vi "Scan1762ARP.vi"() -> ()   [LabVIEW 2012]
uses:
  <vilib>/Utility/file.llb/Write To Spreadsheet File (DBL).vi
panel:
  in  "1762 Sweep freq Span(Hz)":dbl=100000.0
  out "DARK?":i32(graph)=41
  out "Counts":i32=41
  out "DARK?":bool
  out "PMT Counts":i32(graph)=29
  in  "PMT sample time":dbl=0.02
  out "Counts after 1762":i32=29
  out "OuterLoop":i32
  out "InnerLoop":i32=23
  out "Bright Events":dbl=71.0
  in  "Discriminator Level\n (Bright/Dark)":i32=12
  in  "1762 Sweep time (ms)":i32=20
  in  "Comment":string="SPAOM, DPAOM = 83 MHz"
  in  "Rerun BG Every\nnth freq point":dbl=2.0
  in  "PMT sample time":dbl=0.02
  out "Counts finding bright ion":dbl=41.0
  in  "BG Cutoff Limit":dbl=25.0
  in  "Runs per data point":dbl=100.0
  in  "Low Freq":dbl(slide)=82000000.0 min=50000000.0 max=120000000.0 step=1000.0 scale=75000000.0..90000000.0 scale format="%#.5f"
  in  "High Freq":dbl(slide)=85000000.0 min=50000000.0 max=120000000.0 step=1000.0 scale=80000000.0..90000000.0 scale format="%#.0f"
  out "Cur Freq":dbl=85000000.0 format="%#_8f"
  out "Path":path=path "c:/data/1762 Scans/2014-06-11_11-58-27_1762scanWithPumping.txt"
  out "Frequency Scan":cluster{dbl, dbl}[](graph)=[{88000000.0, 1.29}, {87600000.0, 1.0}, {87200000.0, 1.0}, {86800000.0, 1.0}, {86400000.0, 1.0}, {86000000.0, 0.99}, {85600000.0, 1.0}, {85200000.0, 1.0}, {84800000.0, 1.0}, {84400000.0, 0.99}, {84000000.0, 1.0}, {83600000.0, 1.0}, {83200000.0, 0.99}, {82800000.0, 0.88}, {82400000.0, 1.0}, {82000000.0, 1.0}]
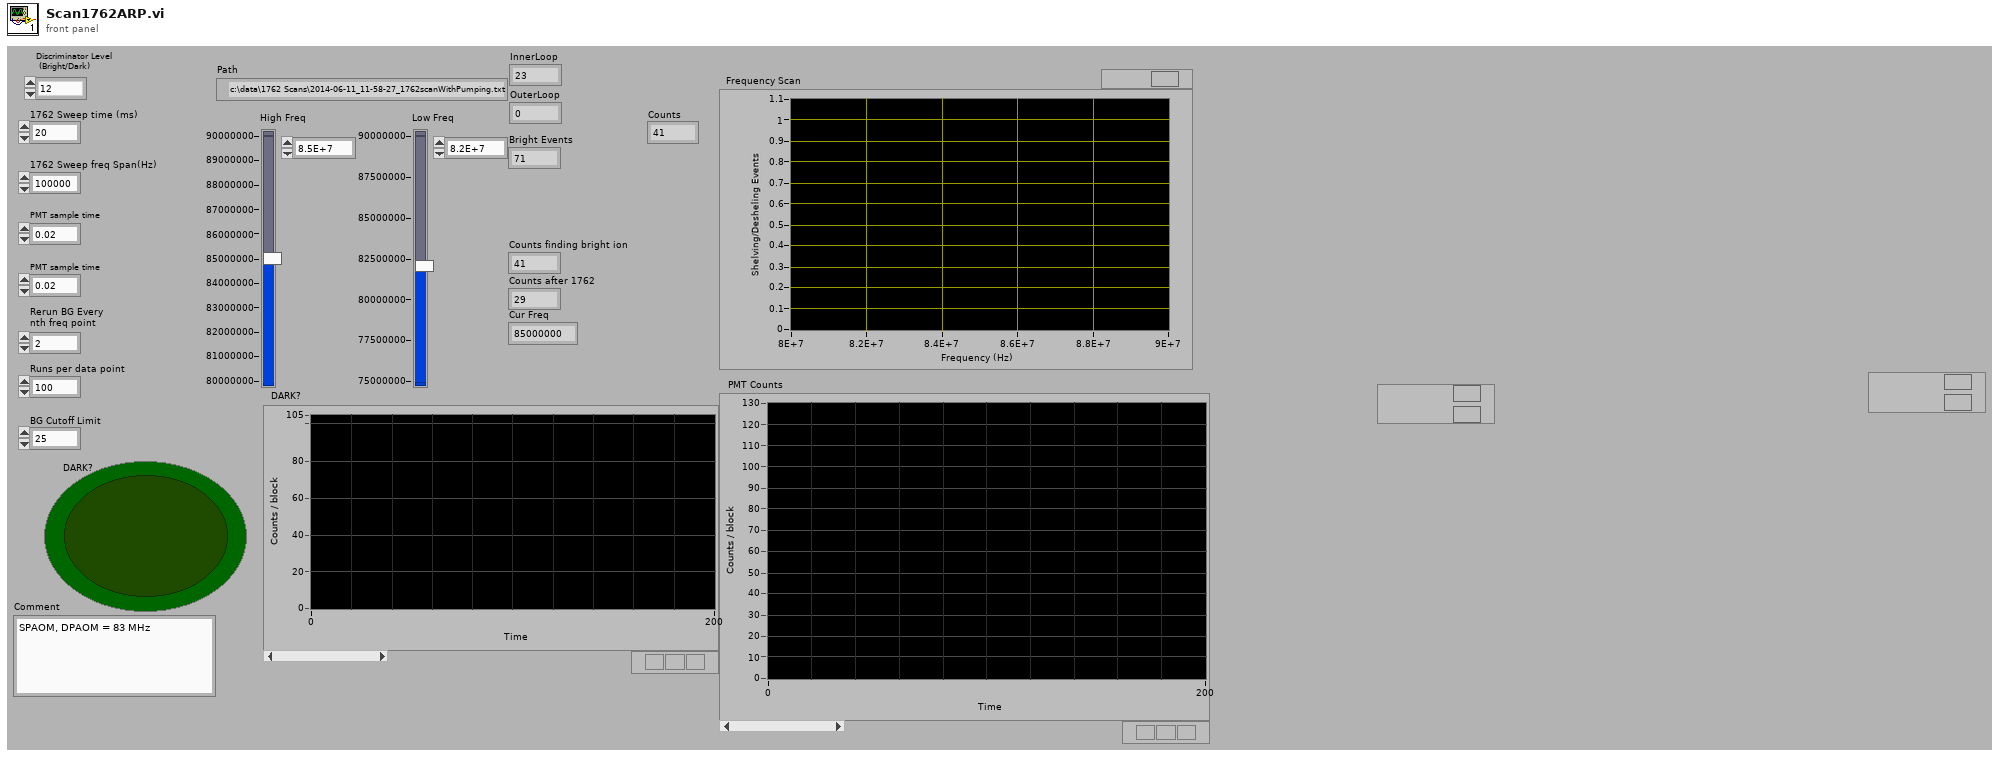
[diagram p1: front panel]
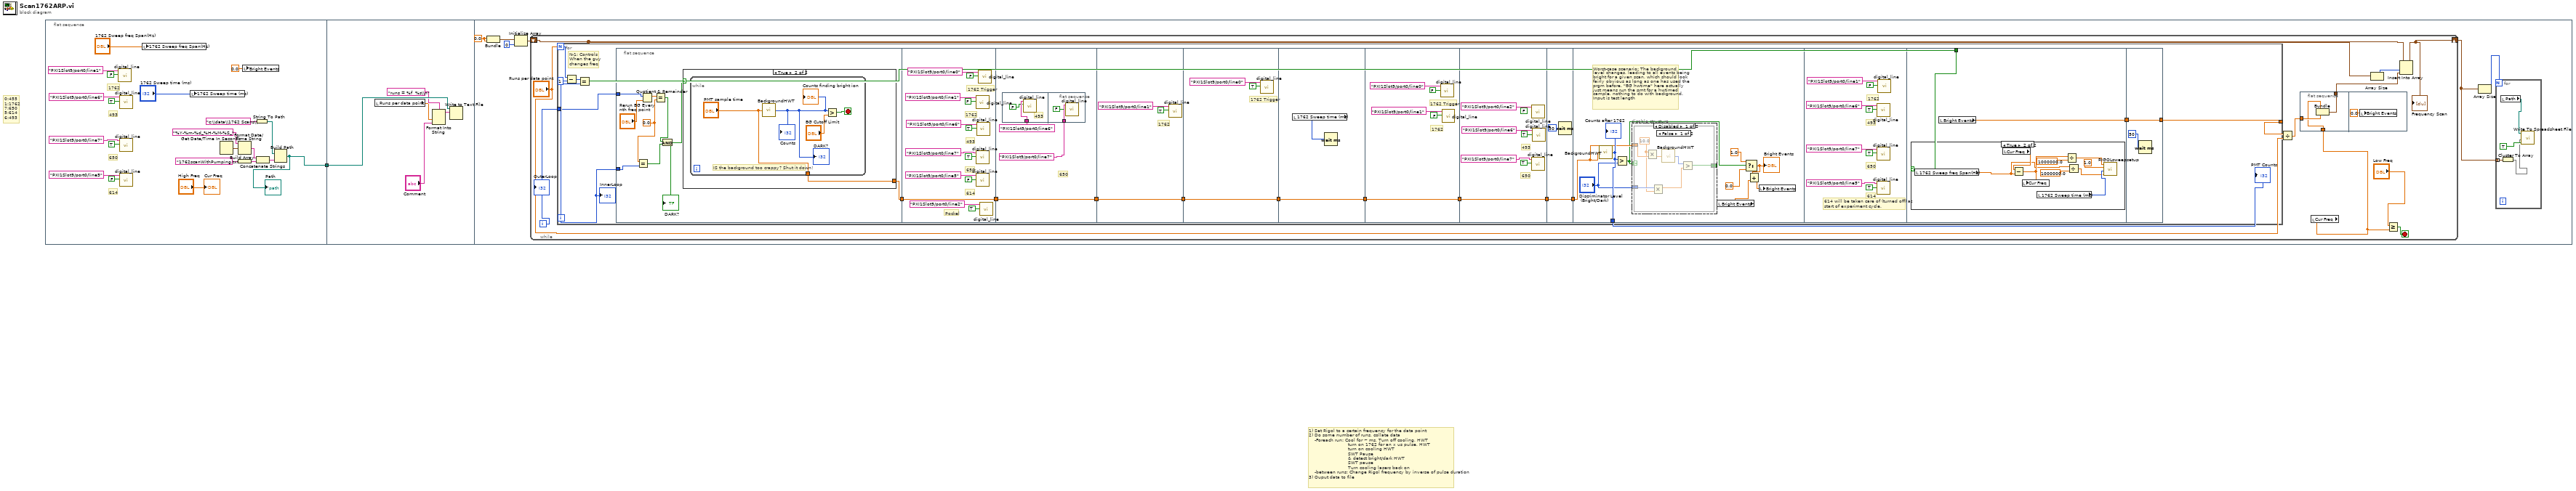
[diagram p0: block diagram]
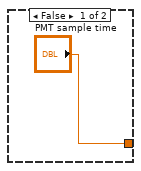
[diagram p2: hidden frame]
diagram:
  # "0:455\n1:1762\n7:650\n5:614\n6:493"
  # "1) Set Rigol to a certain frequency for the data point\n2) Do some number of runs, collate data\n    -Foreach run: Cool for ~ ms, Turn off cooling, HWT\n                           turn on 1762 for an x us pulse, HWT\n                           turn on cooling HWT\n                           SWT Pause\n                           & detect bright/dark HWT\n                           SWT pause\n                           Turn cooling lasers back on \n    -between runs: Change Rigol frequency by inverse of pulse duration\n3) Ouput data to file"
  n1 = flat-sequence {
    tunnel: [w14] -> w1
    tunnel: w1 -> [w27]
    frame #0 {
      # "614"
      # "650"
      # "493"
      # "1762"
      n2 = call "digital_line.vi"("Boolean"=FALSE, "lines"=tag "PXI1Slot9/port0/line1") -> ()  [unwired: 5 in, 1 out]
      n3 = call "digital_line.vi"("Boolean"=TRUE, "lines"=tag "PXI1Slot9/port0/line6") -> ()  [unwired: 5 in, 1 out]
      n4 = call "digital_line.vi"("Boolean"=TRUE, "lines"=tag "PXI1Slot9/port0/line7") -> ()  [unwired: 5 in, 1 out]
      n5 = call "digital_line.vi"("Boolean"=FALSE, "lines"=tag "PXI1Slot9/port0/line5") -> ()  [unwired: 5 in, 1 out]
      n6 = local write "1762 Sweep freq Span(Hz)"("1762 Sweep freq Span(Hz)") -> ()
      n7 = local write "1762 Sweep time (ms)"("1762 Sweep time (ms)") -> ()
      n8 = Get Date/Time In Seconds() -> (seconds since 1Jan1904=w16:timestamp)
      n9 = Format Date/Time String(time format string (%c)="%Y-%m-%d_%H-%M-%S_", seconds (now)=w16) -> (date/time string=w18:string)  [unwired: 1 in]
      n10 = Build Array("1762scanWithPumping.txt") -> (w21:string[])
      n11 = local write "Bright Events"(0.0 ("Bright Events")) -> ()
      n12 = String To Path(string="c:\\data\\1762 Scans\\") -> (path=w22:path)
      n13 = Concatenate Strings(w18, w21) -> (w20:string)
      n14 = Build Path(base path=w22, name or relative path=w20) -> (appended path=w14:path)
      "Path" <- w14
      "Cur Freq" <- "High Freq"
    }
    frame #1 {
      n15 = local read "Runs per data point"() -> (w24:dbl)
      n16 = Format Into String(format string="runs = %f  %s\\n", w24, "Comment") -> (resulting string=w25:string)  [unwired: 2 in, 1 out]
      n17 = Write to Text File(file (use dialog)=w27, text=w25) -> ()  [unwired: 2 in, 3 out]
    }
    frame #2 {
      w32 = 0.0
      n18 = Bundle(w32, w32) -> (w33:cluster{dbl, dbl})  [unwired: 1 in]
      n19 = Initialize Array(w33, 0) -> (w30:cluster{dbl, dbl}[])
      n20 = while {
        shift-right: [w44] -> w28
        shift-left: w30 -> [w45]
        i -> [w43]
        stop <- w47 stop-if-true
        n21 = for {
          N: "Runs per data point" -> [w67]
          tunnel: [w66] -> w40
          tunnel: w43 -> [w63]
          i -> [w64]
          # "N-1: Controls\nWhen the guy\nchanges freq"
          n22 = Subtract(x=w67, y=1) -> (x-y=w70:i32)
          n23 = Equal?(x=w70, y=w64) -> (x = y?=w68:bool)
          n24 = flat-sequence {
            tunnel: w64 -> [w77]
            tunnel: w63 -> [w72]
            tunnel: [w71] -> w61
            tunnel: w61 -> [w98]
            tunnel: [w98] -> w60
            tunnel: [w101] -> w59
            tunnel: w60 -> [w101]
            tunnel: w59 -> [w108]
            tunnel: [w108] -> w58
            tunnel: [w111] -> w56
            tunnel: w58 -> [w111]
            tunnel: w56 -> [w113]
            tunnel: [w113] -> w55
            tunnel: w55 -> [w118]
            tunnel: [w118] -> w57
            tunnel: w57 -> [w124]
            tunnel: [w124] -> w54
            tunnel: w54 -> [w126]
            tunnel: [w126] -> w53
            tunnel: w53 -> [w129]
            tunnel: [w130] -> w62
            tunnel: w68 -> [w156]
            tunnel: [w157] -> w65
            tunnel: [w168] -> w66
            tunnel: w65 -> [w168]
            frame #0 {
              w76 = 0.0 ("x")
              n25 = Equal?(x=w76, y=w77) -> (x = y?=w74:bool)
              n26 = Quotient & Remainder(x=w72, y="Rerun BG Every\nnth freq point") -> (x-y*floor(x/y)=w78:dbl)  [unwired: 1 out]
              n27 = Equal?(x=w78, y=w76) -> (x = y?=w75:bool)
              n28 = And(x=w75, y=w74) -> (x .and. y?=w73:bool)
              "DARK?" <- w73
              n29 = case shown="True" w73 {
                tunnel: ["PMT sample time" w81] -> w71
                frame False {
                }
                frame True {
                  n30 = while {
                    tunnel: ["PMT sample time"] -> w81
                    stop <- w84 stop-if-true
                    # "IS the background too crappy? Shut it down!"
                    n31 = call "BackgroundHWT.vi"("Sample Time(seconds)"="PMT sample time") -> ("Counts"=w82:i32)
                    "Counts finding bright ion" <- w82
                    "Counts" <- w82
                    "DARK?" <- w82
                    n32 = Greater?(x=w82, y="BG Cutoff Limit") -> (0:w84:bool)
                  }
                }
              }
            }
            frame #1 {
              # "Pockel"
              # "1762 Trigger"
              # "614"
              # "650"
              # "493"
              # "1762"
              n33 = call "digital_line.vi"("Boolean"=FALSE, "lines"=tag "PXI1Slot9/port0/line1") -> ()  [unwired: 5 in, 1 out]
              n34 = call "digital_line.vi"("Boolean"=TRUE, "lines"=tag "PXI1Slot9/port0/line7") -> ()  [unwired: 5 in, 1 out]
              n35 = call "digital_line.vi"("Boolean"=FALSE, "lines"=tag "PXI1Slot9/port0/line5") -> ()  [unwired: 5 in, 1 out]
              n36 = call "digital_line.vi"("Boolean"=TRUE, "lines"=tag "PXI1Slot9/port0/line6") -> ()  [unwired: 5 in, 1 out]
              n37 = call "digital_line.vi"("Boolean"=FALSE, "lines"=tag "PXI1Slot9/port0/line0") -> ()  [unwired: 5 in, 1 out]
              n38 = call "digital_line.vi"("Boolean"=TRUE, "lines"=tag "PXI1Slot9/port0/line2") -> ()  [unwired: 5 in, 1 out]
            }
            frame #2 {
              # "650"
              n39 = flat-sequence {
                tunnel: tag "PXI1Slot9/port0/line6" ("lines") -> [w103]
                tunnel: tag "PXI1Slot9/port0/line7" ("lines") -> [w105]
                frame #0 {
                  # "493"
                  n40 = call "digital_line.vi"("Boolean"=FALSE, "lines"=w103) -> ()  [unwired: 5 in, 1 out]
                }
                frame #1 {
                  n41 = call "digital_line.vi"("Boolean"=FALSE, "lines"=w105) -> ()  [unwired: 5 in, 1 out]
                }
              }
            }
            frame #3 {
              # "1762"
              n42 = call "digital_line.vi"("Boolean"=TRUE, "lines"=tag "PXI1Slot9/port0/line1") -> ()  [unwired: 5 in, 1 out]
            }
            frame #4 {
              # "1762 Trigger"
              n43 = call "digital_line.vi"("Boolean"=TRUE, "lines"=tag "PXI1Slot9/port0/line0") -> ()  [unwired: 5 in, 1 out]
            }
            frame #5 {
              n44 = local read "1762 Sweep time (ms)"() -> (w112:i32)
              n45 = Wait (ms)(milliseconds to wait=w112) -> ()  [unwired: 1 out]
            }
            frame #6 {
              # "1762 Trigger"
              # "1762"
              n46 = call "digital_line.vi"("Boolean"=FALSE, "lines"=tag "PXI1Slot9/port0/line0") -> ()  [unwired: 5 in, 1 out]
              n47 = call "digital_line.vi"("Boolean"=FALSE, "lines"=tag "PXI1Slot9/port0/line1") -> ()  [unwired: 5 in, 1 out]
            }
            frame #7 {
              (unwired) FALSE
              # "650"
              # "493"
              n48 = call "digital_line.vi"("lines"=tag "PXI1Slot9/port0/line2") -> ()  [unwired: 6 in, 1 out]
              n49 = call "digital_line.vi"("Boolean"=TRUE, "lines"=tag "PXI1Slot9/port0/line7") -> ()  [unwired: 5 in, 1 out]
              n50 = call "digital_line.vi"("Boolean"=TRUE, "lines"=tag "PXI1Slot9/port0/line6") -> ()  [unwired: 5 in, 1 out]
            }
            frame #8 {
              n51 = Wait (ms)(milliseconds to wait=u32 50) -> ()  [unwired: 1 out]
            }
            frame #9 {
              # "Worst-case scenario: The background\nlevel changes, leading to all events being\nbright for a given scan, which should look\nfairly obvious as long as one has used the\nprgm before. \"BG hwtime\" here actually\njust means run the pmt for a hwtimed\nsample, nothing to do with background.\nInput is test length"
              n52 = call "BackgroundHWT.vi"("Sample Time(seconds)"=w129) -> ("Counts"=w130:i32)
              "Counts after 1762" <- w130
              n53 = Greater?(x=w130, y="Discriminator Level\n (Bright/Dark)") -> (0:w127:bool)
              n54 = disable-structure shown="Disabled" {
                disable-tunnel: w129 -> [w139 _]
                disable-tunnel: "Discriminator Level\n (Bright/Dark)" -> [w138 _]
                disable-tunnel: w127 -> [w137 _]
                disable-tunnel: [w136 _] -> _
                frame Disabled {
                  n55 = case shown="False" w137 {
                    selector: w137 -> [_ w147]
                    tunnel: w139 -> [w146 _]
                    tunnel: w138 -> [w143 _]
                    tunnel: [w140 w147] -> w136
                    frame False {
                      w141 = 10.0 ("x")
                      n56 = Multiply(x=w141, y=w146) -> (x*y=w145:dbl)
                      n57 = Multiply(x=w143, y=w141) -> (x*y=w142:dbl)
                      n58 = call "BackgroundHWT.vi"("Sample Time(seconds)"=w145) -> ("Counts"=w144:i32)
                      n59 = Greater?(x=w144, y=w142) -> (0:w140:bool)
                    }
                    frame True {
                    }
                  }
                }
                frame Enabled {
                }
              }
              n60 = local read "Bright Events"() -> (w131:dbl)
              n61 = Select(t=1.0, s=w127, f=0.0) -> (s? t:f=w133:dbl)
              "Bright Events" <- w133
              n62 = Add(x=w133, y=w131) -> (x+y=w132:dbl)
              n63 = local write "Bright Events"(w132) -> ()
            }
            frame #10 {
              # "614 will be taken care of (turned off) at\nstart of experiment cycle."
              # "614"
              # "650"
              # "493"
              # "1762"
              n64 = call "digital_line.vi"("Boolean"=TRUE, "lines"=tag "PXI1Slot9/port0/line6") -> ()  [unwired: 5 in, 1 out]
              n65 = call "digital_line.vi"("Boolean"=TRUE, "lines"=tag "PXI1Slot9/port0/line7") -> ()  [unwired: 5 in, 1 out]
              n66 = call "digital_line.vi"("Boolean"=TRUE, "lines"=tag "PXI1Slot9/port0/line5") -> ()  [unwired: 5 in, 1 out]
              n67 = call "digital_line.vi"("Boolean"=FALSE, "lines"=tag "PXI1Slot9/port0/line1") -> ()  [unwired: 5 in, 1 out]
            }
            frame #11 {
              n68 = case shown="True" w156 {
                frame False {
                }
                frame True {
                  n69 = local read "1762 Sweep freq Span(Hz)"() -> (w159:dbl)
                  n70 = local read "Cur Freq"() -> (w166:dbl)
                  n71 = Subtract(x=w166, y=w159) -> (x-y=w165:dbl)
                  n72 = local write "Cur Freq"(w165) -> ()
                  n73 = local read "1762 Sweep time (ms)"() -> (w162:i32)
                  n74 = Divide(x=w165, y=1000000.0) -> (x/y=w161:dbl)
                  n75 = Divide(x=w159, y=1000000.0) -> (x/y=w158:dbl)
                  n76 = call "RIGOLsweepsetup.vi"("AP Sweep Width (MHz)"=w158, "Time (ms)"=w162, "Amplitude (Vpp)"=1.0, "Frequency (MHz)"=w161) -> ()  [unwired: 8 in]
                }
              }
              n77 = local read "Bright Events"() -> (w157:dbl)
            }
            frame #12 {
              n78 = Wait (ms)(milliseconds to wait=u32 50) -> ()  [unwired: 1 out]
            }
          }
          "InnerLoop" <- w64
          "PMT Counts" <- w62
        }
        n79 = Divide(x=w40, y="Runs per data point") -> (x/y=w39:dbl)
        n80 = flat-sequence {
          tunnel: w39 -> [w51]
          tunnel: [w50] -> w42
          tunnel: w41 -> [w49]
          frame #0 {
            n81 = Bundle("Cur Freq"=w49, w51) -> (w50:cluster{"Cur Freq":dbl, dbl})  [unwired: 1 in]
          }
          frame #1 {
            n82 = local write "Bright Events"(0.0 ("Bright Events")) -> ()
          }
        }
        n83 = local read "Cur Freq"() -> (w41:dbl)
        n84 = Array Size(array=w45) -> (size(s)=w46:i32)
        n85 = Greater Or Equal?(x="Low Freq", y=w41) -> (x >= y?=w47:bool)
        n86 = Insert Into Array(array=w45, index=w46, new element=w42) -> (w44:cluster{dbl, dbl}[])
        "Frequency Scan" <- w44
        "OuterLoop" <- w43
      }
      n87 = Array Size(array=w28) -> (size(s)=w29:i32)
      n88 = for {
        N: w29 -> [_]
        tunnel: w28 -> [w37] mode=indexing
        n89 = local read "Path"() -> (w34:path)
        n90 = Cluster To Array(cluster=w37) -> (array=w35:dbl[])
        n91 = call-poly <vilib>:"Write To Spreadsheet File.vi"("append to file? (new file:F)"=TRUE, "1D data"=w35, "file path (dialog if empty)"=w34) -> ()  [unwired: 5 in, 1 out]
      }
    }
  }
